vi "trapezoid-profile-position-ctrl.vi"() -> ()   [LabVIEW 2019]
uses:
  <vilib>/Rock Robotics/WPI/ThirdParty/JAS_Junk/TrajLib/TrapProfile_Calculate.vi
  <vilib>/Rock Robotics/WPI/ThirdParty/JAS_Junk/TrajLib/TrapProfile_New.vi
  <vilib>/Rock Robotics/WPI/ThirdParty/JAS_Junk/TrajLib/TrapProfile_TotalTime.vi
  <vilib>/Rock Robotics/WPI/ThirdParty/JAS_Junk/TrajLib/TrapProfConstraint_New.vi
  <vilib>/Rock Robotics/WPI/ThirdParty/JAS_Junk/TrajLib/TrapProfState_New.vi
  <vilib>/Rock Robotics/WPI/ThirdParty/JAS_Junk/TrajLib/TrapProfile_IsFinished.vi
  <vilib>/Rock Robotics/WPI/ThirdParty/JAS_Junk/TrajLib/TrapProfile_Direct.vi
  <vilib>/Rock Robotics/WPI/ThirdParty/JAS_Junk/TrajLib/TrapProfile_ShouldFlipAcceleration.vi
  <vilib>/Rock Robotics/SystemInterfaces/NetworkCommunication/NetComm_UsageReport_report.vi
  <vilib>/addons/control/pid/pid.llb/PID Lead-Lag (DBL).vi
  <vilib>/Rock Robotics/WPI/ThirdParty/JAS_Junk/TrajLib/Globals/Util_LibraryGlobals.vi
  <vilib>/addons/control/pid/NI_PID_pid.lvlib
  <vilib>/Rock Robotics/WPI/ThirdParty/JAS_Junk/TrajLib/Trajectory_Library.lvlib
panel:
  in  "Tab Control":T1(tab)
  in  "Desired Position":dbl(slide) min=0.0 max=90.0 scale=0.0..90.0
  in  "Auto - Set Position To 0 / Manual - Lower":bool
  in  "Auto - Set Position to 90 / Manual - Raise":bool
  in  "Set Position to Desired\n(Select to activate position)":bool
  out "Selected Setpoint \n(In Manual \ntracks Position)":dbl
  out "Current Position 2":dbl format="%.2f"
  out "Motor Demand":dbl format="%#.2f"
  out "Position Error":dbl format="%#3.2f"
  out "SP, PV, CO Chart":T2(graph)
  out "Current Position":dbl(knob) scale=-10.0..100.0
  in  "Auto / Manual":bool=TRUE
  in  "MinLimitSwitch":bool
  in  "MaxLimitSwitch":bool
  out "In Position":bool
  in  "Max Accel":dbl=6.0 format="%#_13g"
  out "Current-Setpoint":dbl
  out "Current-Position":dbl
  out "Manual-Lower":bool
  out "Manual-Raise":bool
  out "Motor-Demand":dbl
  # "Example of Closed Loop Position Control Using a Motor\n(Simple Example 002)"
  # "This example adds a \"Manual\" mode so that the arm\ncan still be moved if the position indication fails.\nThis example also adds failsafe min and max positions\nand optional inputs from limit switches to stop the motor \nfrom traveling too far."
  # "This value shows the error between the current position\nand the desired position."
  # "This value shows the current position.  This is measured by an encoder, a potentiometer, or some other sensor.  This is called the \"Process Variable\","
  # "Press one of the buttons to set the desired \nposition.  This \"target\" value is called\nthe \"Set Point\".  In \"Manual\" mode hold the 0 or 90 button\ndown to manually run the motor."
  # "This value shows the current motor output demand.  This\ncould also be a motor speed demand and another closed\nloop controller would control the motor speed.  In this simple\nexample this value is used to drive the simulated motor directly.\nThis motor demand is called the \"Control Output\"."
  # "The action caused by the motor causes the position to change."
  # "Toggle these switches to simulate a limit switch input."
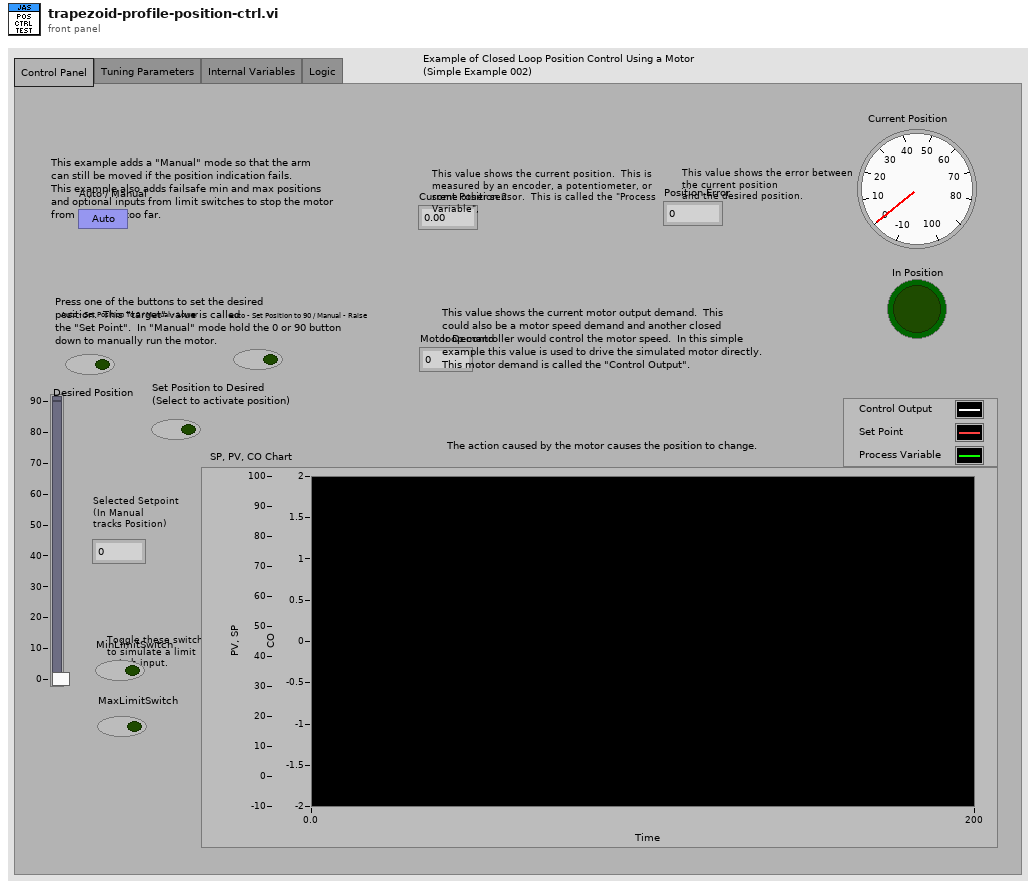
[diagram p1: front panel]
types:
  T1 = enum32{"Control Panel", "Tuning Parameters", "Internal Variables", "Logic"}
  T2 = cluster{"MotorDemand":dbl, "CurrentSetpoint":dbl, "CurrentPosition":dbl}
  T3 = cluster{"gain":dbl, "lag time":dbl, "lead time":dbl}
  T4 = cluster{"Motor-Demand":dbl, "Current-Setpoint":dbl, "Current-Position":dbl}
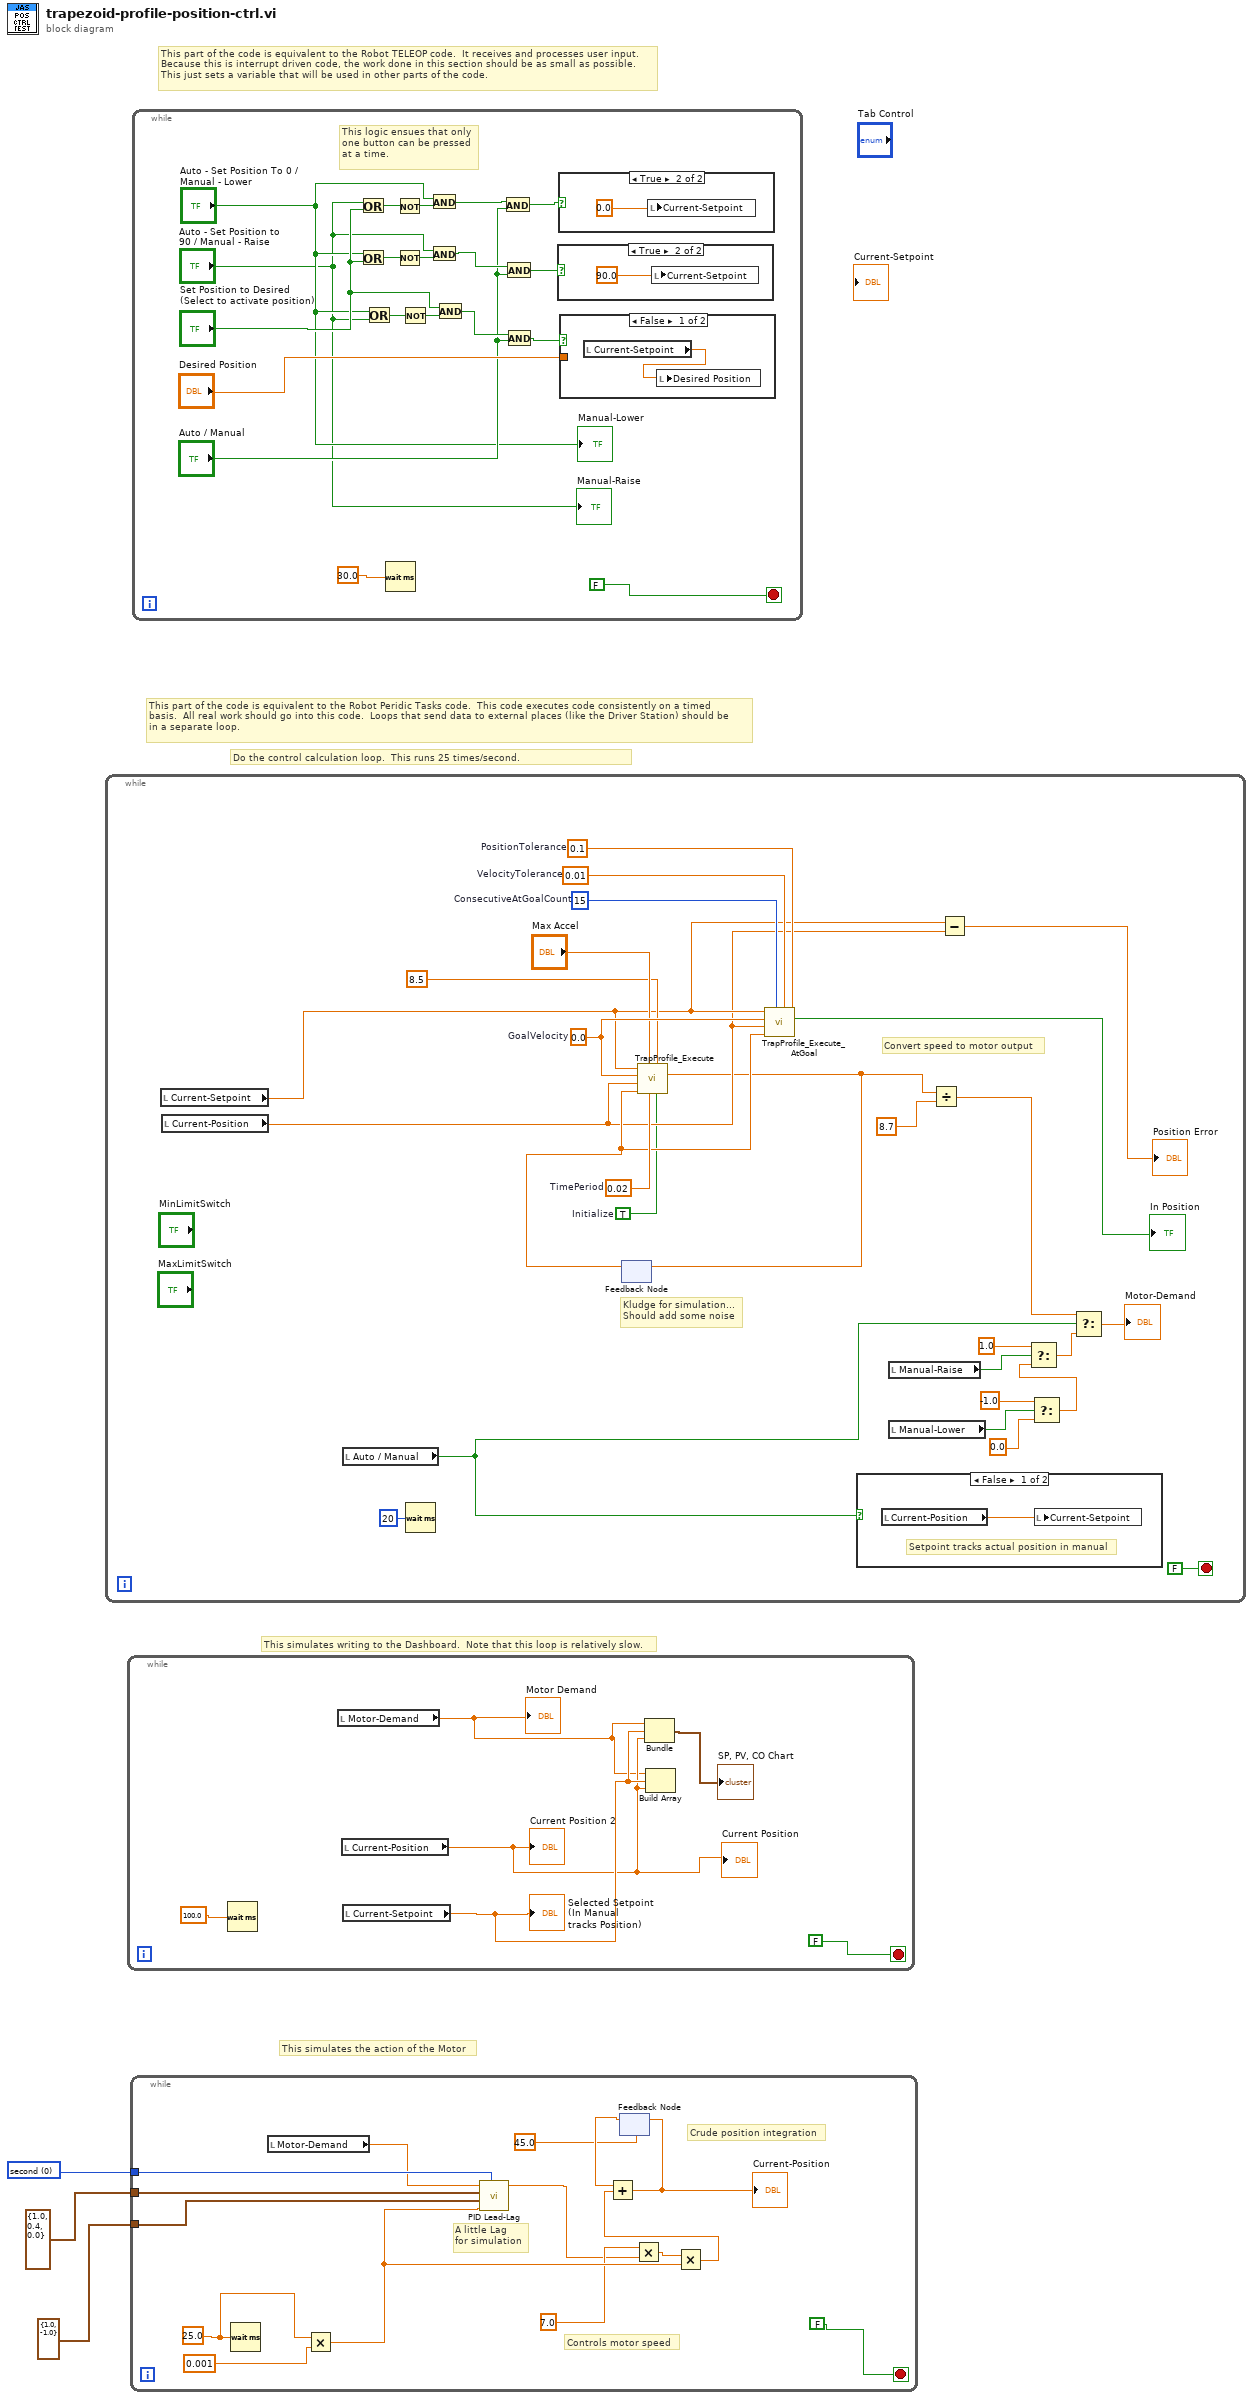
[diagram p0: block diagram]
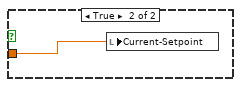
[diagram p3: hidden frame]
diagram:
  w3 = u16 0 items=["second", "minute"] ("time unit")
  # "This simulates the action of the Motor"
  # "This simulates writing to the Dashboard.  Note that this loop is relatively slow."
  # "Do the control calculation loop.  This runs 25 times/second."
  # "This part of the code is equivalent to the Robot Peridic Tasks code.  This code executes code consistently on a timed\nbasis.  All real work should go into this code.  Loops that send data to external places (like the Driver Station) should be \nin a separate loop."
  # "This part of the code is equivalent to the Robot TELEOP code.  It receives and processes user input.\nBecause this is interrupt driven code, the work done in this section should be as small as possible.\nThis just sets a variable that will be used in other parts of the code."
  n1 = while {
    stop <- FALSE stop-if-true
    w19 = 15  # ConsecutiveAtGoalCount
    w18 = 0.01  # VelocityTolerance
    w17 = 0.1  # PositionTolerance
    w20 = 0.0  # GoalVelocity
    w15 = 0.02  # TimePeriod
    w4 = TRUE  # Initialize
    # "Convert speed to motor output"
    # "Kludge for simulation...\nShould add some noise"
    n2 = local read "Current-Setpoint"() -> (w12:dbl)
    n3 = local read "Current-Position"() -> (w8:dbl)
    n4 = local read "Auto / Manual"() -> (w25:bool)
    n5 = Wait (ms)(milliseconds to wait=u32 20) -> ()  [unwired: 1 out]
    n6 = feedback #1() -> (w9:dbl)  [unwired: 1 in]
    n7 = call <vilib>:"TrapProfile_Execute.vi"("Initialize"=w4, "Max Speed"=8.5, "TimePeriod"=w15, "Max Accel"="Max Accel", "CurrentVelocity"=w9, "CurrentPosition"=w8, "GoalVelocity"=w20, "GoalPosition"=w12) -> ("VelocityDmd"=w5:dbl)  [unwired: 3 out]
    n8 = feedback-in #1(w5) -> ()
    n9 = call <vilib>:"TrapProfile_Execute_AtGoal.vi"("PositionTolerance"=w17, "VelocityTolerance"=w18, "ConsecutiveAtGoalCount"=w19, "CurrentVelocity"=w9, "CurrentPosition"=w8, "GoalVelocity"=w20, "GoalPosition"=w12) -> ("AtGoal"=→"In Position":bool)  [unwired: 4 in]
    n10 = case shown="False" w25 {
      frame False {
        # "Setpoint tracks actual position in manual"
        n11 = local read "Current-Position"() -> (w31:dbl)
        n12 = local write "Current-Setpoint"(w31) -> ()
      }
      frame True {
      }
    }
    n13 = local read "Manual-Raise"() -> (w24:bool)
    n14 = local read "Manual-Lower"() -> (w23:bool)
    n15 = Divide(x=w5, y=8.7) -> (x/y=w6:dbl)
    n16 = Subtract(x=w12, y=w8) -> (x-y=→"Position Error":dbl)
    n17 = Select(t=-1.0, s=w23, f=0.0) -> (s? t:f=w27:dbl)
    n18 = Select(t=1.0, s=w24, f=w27) -> (s? t:f=w26:dbl)
    n19 = Select(t=w6, s=w25, f=w26) -> (s? t:f=→"Motor-Demand":dbl)
  }
  n20 = while {
    stop <- FALSE stop-if-true
    n21 = Wait (ms)(milliseconds to wait=100.0) -> ()  [unwired: 1 out]
    n22 = local read "Motor-Demand"() -> (w32:dbl)
    "Motor Demand" <- w32
    n23 = local read "Current-Position"() -> (w33:dbl)
    "Current Position 2" <- w33
    "Current Position" <- w33
    n24 = local read "Current-Setpoint"() -> (w34:dbl)
    "Selected Setpoint \n(In Manual \ntracks Position)" <- w34
    n25 = Bundle("Motor-Demand"=w32, "Current-Setpoint"=w34, "Current-Position"=w33) -> (→"SP, PV, CO Chart":T4)  [unwired: 1 in]
    n26 = Build Array(w32, w34, w33) -> ()  [unwired: 1 out]
  }
  n27 = while {
    tunnel: w3 -> [w52]
    tunnel: T3 {"gain"=1.0, "lag time"=0.4, "lead time"=0.0} ("tuning parameters") -> [w51]
    tunnel: cluster{"output high":dbl, "output low":dbl} {"output high"=1.0, "output low"=-1.0} ("output range") -> [w49]
    stop <- FALSE stop-if-true
    w41 = 25.0
    # "Controls motor speed"
    # "Crude position integration"
    # "A little Lag\nfor simulation"
    n28 = Wait (ms)(milliseconds to wait=w41) -> ()  [unwired: 1 out]
    n29 = local read "Motor-Demand"() -> (w38:dbl)
    n30 = Multiply(x=w41, y=0.001) -> (x*y=w48:dbl)
    n31 = call-poly <vilib>:"PID Lead-Lag.vi"("time unit"=w52, "dt (s)"=w48, "output range"=w49, "tuning parameters"=w51, "input"=w38) -> ("output"=w40:dbl)  [unwired: 3 in, 1 out]
    n32 = feedback #2(45.0) -> (w46:dbl)
    n33 = Multiply(x=7.0, y=w40) -> (x*y=w47:dbl)
    n34 = Multiply(x=w47, y=w48) -> (x*y=w44:dbl)
    n35 = Add(x=w46, y=w44) -> (x+y=w39:dbl)
    "Current-Position" <- w39
    n36 = feedback-in #2(w39) -> ()
  }
  n37 = while {
    stop <- FALSE stop-if-true
    # "This logic ensues that only\none button can be pressed\nat a time."
    n38 = Or(x="Auto - Set Position to 90 / Manual - Raise", y="Set Position to Desired\n(Select to activate position)") -> (x .or. y?=w71:bool)
    n39 = Or(x="Auto - Set Position To 0 / Manual - Lower", y="Set Position to Desired\n(Select to activate position)") -> (x .or. y?=w69:bool)
    n40 = Or(x="Auto - Set Position To 0 / Manual - Lower", y="Auto - Set Position to 90 / Manual - Raise") -> (x .or. y?=w67:bool)
    n41 = Wait (ms)(milliseconds to wait=30.0) -> ()  [unwired: 1 out]
    n42 = Not(x=w71) -> (.not. x?=w70:bool)
    n43 = Not(x=w69) -> (.not. x?=w68:bool)
    n44 = Not(x=w67) -> (.not. x?=w66:bool)
    n45 = And(x="Auto - Set Position To 0 / Manual - Lower", y=w70) -> (x .and. y?=w61:bool)
    n46 = And(x="Auto - Set Position to 90 / Manual - Raise", y=w68) -> (x .and. y?=w57:bool)
    n47 = And(x="Set Position to Desired\n(Select to activate position)", y=w66) -> (x .and. y?=w56:bool)
    n48 = And(x=w61, y="Auto / Manual") -> (x .and. y?=w60:bool)
    n49 = And(x=w57, y="Auto / Manual") -> (x .and. y?=w59:bool)
    n50 = And(x=w56, y="Auto / Manual") -> (x .and. y?=w58:bool)
    n51 = case shown="True" w59 {
      frame False {
      }
      frame True {
        n52 = local write "Current-Setpoint"(90.0) -> ()
      }
    }
    n53 = case shown="True" w60 {
      frame False {
      }
      frame True {
        n54 = local write "Current-Setpoint"(0.0) -> ()
      }
    }
    n55 = case shown="False" w58 {
      tunnel: "Desired Position" -> [_ w73]
      frame False {
        n56 = local read "Current-Setpoint"() -> (w72:dbl)
        n57 = local write "Desired Position"(w72) -> ()
      }
      frame True {
        n58 = local write "Current-Setpoint"(w73) -> ()
      }
    }
    "Manual-Raise" <- "Auto - Set Position to 90 / Manual - Raise"
    "Manual-Lower" <- "Auto - Set Position To 0 / Manual - Lower"
  }
